vi "svx_Oct_Waterfall Shortcut Menu.vi"(7 "main graph?":bool, 9 "Container State":T2, 10 "State":T1, 11 "menu reference in":refnum<k9>) -> (3 "menu referenceout":refnum<k9>)   [LabVIEW 2017, in "SVX Octave Waterfall Graph.xctl"]
uses:
  <vilib>/addons/_XControls/Octave Waterfall Graph/SVX Octave Waterfall Graph.xctl
  <vilib>/_xctls/Container State.ctl
  <vilib>/addons/_XControls/Octave Waterfall Graph/subVIs/svx_Oct_Waterfall State.ctl
  <vilib>/_xctls/XControlSupport.lvlib
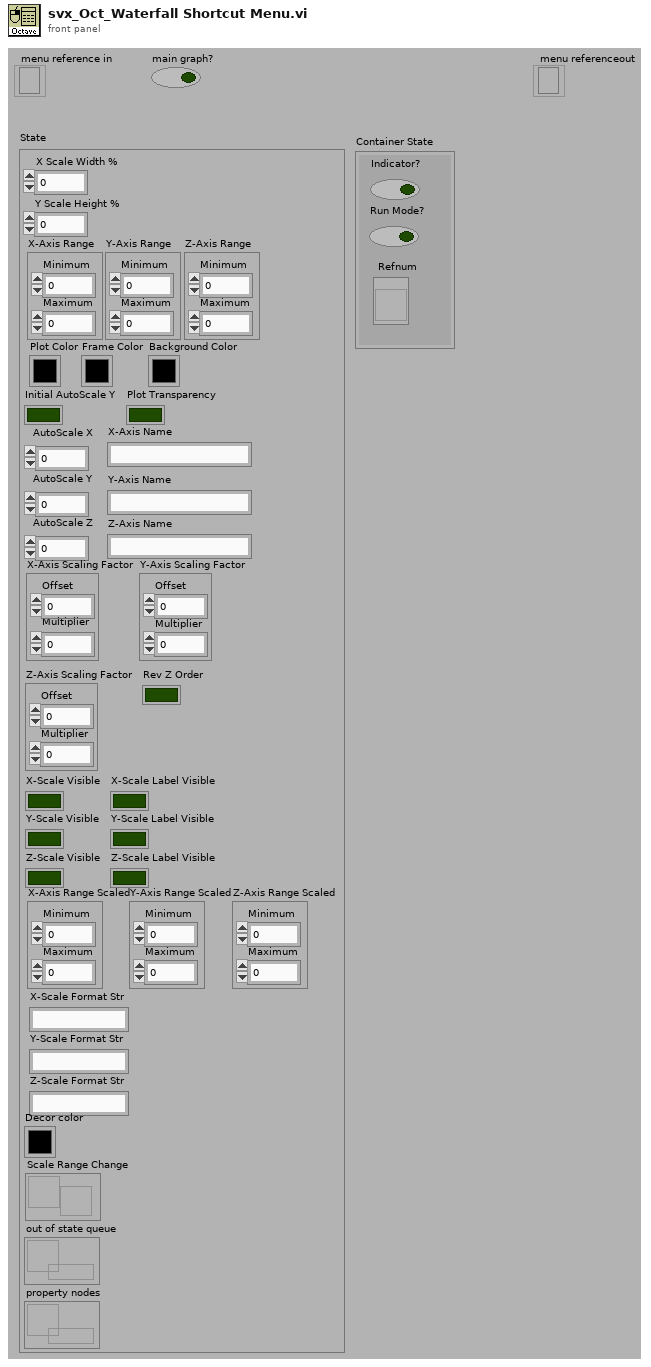
[diagram p1: front panel]
types:
  T1 = typedef "SVX Octave Waterfall Graph.xctl/svx_Oct_Waterfall State.ctl" = cluster{"X Scale Width %":dbl, "Y Scale Height %":dbl, "X-Axis Range":cluster{"Minimum":dbl, "Maximum":dbl}, "Y-Axis Range":cluster{"Minimum":dbl, "Maximum":dbl}, "Z-Axis Range":cluster{"Minimum":dbl, "Maximum":dbl}, "Plot Color":u32, "Frame Color":u32, "Background Color":u32, "Initial AutoScale Y":bool, "AutoScale X":u8, "AutoScale Y":u8, "AutoScale Z":u8, "Plot Transparency":bool, "X-Axis Name":string, "Y-Axis Name":string, "Z-Axis Name":string, "X-Axis Scaling Factor":cluster{"Offset":dbl, "Multiplier":dbl}, "Y-Axis Scaling Factor":cluster{"Offset":dbl, "Multiplier":dbl}, "Z-Axis Scaling Factor":cluster{"Offset":dbl, "Multiplier":dbl}, "X-Scale Visible":bool, "Y-Scale Visible":bool, "Z-Scale Visible":bool, "X-Scale Label Visible":bool, "Y-Scale Label Visible":bool, "Z-Scale Label Visible":bool, "X-Axis Range Scaled":cluster{"Minimum":dbl, "Maximum":dbl}, "Y-Axis Range Scaled":cluster{"Minimum":dbl, "Maximum":dbl}, "Z-Axis Range Scaled":cluster{"Minimum":dbl, "Maximum":dbl}, "Rev Z Order":bool, "X-Scale Format Str":string, "Y-Scale Format Str":string, "Z-Scale Format Str":string, "Decor color":u32, "Scale Range Change":refnum<user-event>, "out of state queue":refnum<queue>, "property nodes":refnum<queue>}
  T2 = typedef "XControlSupport.lvlib/Container State.ctl" = cluster{"Indicator?":bool, "Run Mode?":bool, " Refnum":refnum<vi>}
  T3 = cluster{"menu tag":string, "items to delete":string[], "new menu":cluster{"item names":string, "item tags":string, "after item":string}[], "root?":bool}
  T4 = cluster{"menu tag":string, "items to delete":string[], "new menu":cluster{"item names":string, "item tags":string, "after item":string}[], "root?":bool}[]
  T5 = cluster{"item names":string, "item tags":string, "after item":string}[]
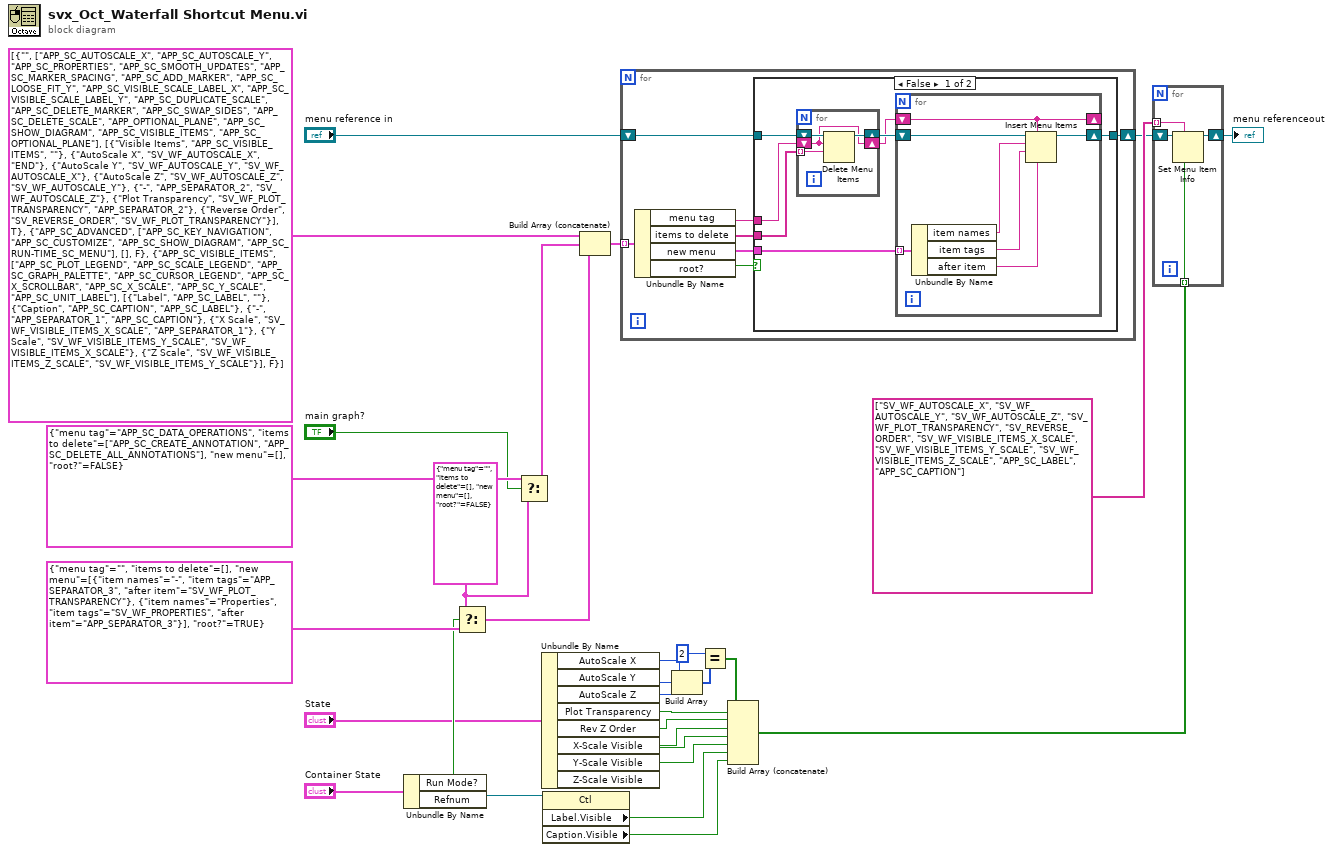
[diagram p0: block diagram]
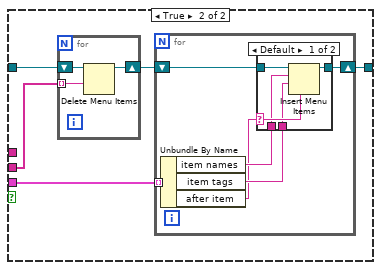
[diagram p2: hidden frame]
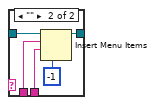
[diagram p3: hidden frame]
diagram:
  w27 = T3 {"menu tag"="", "items to delete"=[], "new menu"=[], "root?"=FALSE} ("t")
  n1 = Unbundle By Name("Container State") -> ("Run Mode?"=w6:bool, "Refnum"=w20:refnum<vi>)
  n2 = Select(t=w27, s=w6, f=T3 {"menu tag"="", "items to delete"=[], "new menu"=[{"item names"="-", "item tags"="APP_SEPARATOR_3", "after item"="SV_WF_PLOT_TRANSPARENCY"}, {"item names"="Properties", "item tags"="SV_WF_PROPERTIES", "after item"="APP_SEPARATOR_3"}], "root?"=TRUE} ("menu item")) -> (s? t:f=w24:T3)
  n3 = Select(t=T3 {"menu tag"="APP_SC_DATA_OPERATIONS", "items to delete"=["APP_SC_CREATE_ANNOTATION", "APP_SC_DELETE_ALL_ANNOTATIONS"], "new menu"=[], "root?"=FALSE} ("menu item"), s="main graph?", f=w27) -> (s? t:f=w25:T3)
  n4 = Unbundle By Name("State") -> ("AutoScale X"=w15:u8, "AutoScale Y"=w16:u8, "AutoScale Z"=w13:u8, "Plot Transparency"=w3:bool, "Rev Z Order"=w2:bool, "X-Scale Visible"=w17:bool, "Y-Scale Visible"=w18:bool, "Z-Scale Visible"=w19:bool)
  n5 = property class="Ctl"(reference=w20) -> ("Label.Visible"=w21:bool, "Caption.Visible"=w22:bool)  [unwired: 1 in, 2 out]
  n6 = Build Array (concatenate)(T4 [{"menu tag"="", "items to delete"=["APP_SC_AUTOSCALE_X", "APP_SC_AUTOSCALE_Y", "APP_SC_PROPERTIES", "APP_SC_SMOOTH_UPDATES", "APP_SC_MARKER_SPACING", "APP_SC_ADD_MARKER", "APP_SC_LOOSE_FIT_Y", "APP_SC_VISIBLE_SCALE_LABEL_X", "APP_SC_VISIBLE_SCALE_LABEL_Y", "APP_SC_DUPLICATE_SCALE", "APP_SC_DELETE_MARKER", "APP_SC_SWAP_SIDES", "APP_SC_DELETE_SCALE", "APP_OPTIONAL_PLANE", "APP_SC_SHOW_DIAGRAM", "APP_SC_VISIBLE_ITEMS", "APP_SC_OPTIONAL_PLANE"], "new menu"=[{"item names"="Visible Items", "item tags"="APP_SC_VISIBLE_ITEMS", "after item"=""}, {"item names"="AutoScale X", "item tags"="SV_WF_AUTOSCALE_X", "after item"="END"}, {"item names"="AutoScale Y", "item tags"="SV_WF_AUTOSCALE_Y", "after item"="SV_WF_AUTOSCALE_X"}, {"item names"="AutoScale Z", "item tags"="SV_WF_AUTOSCALE_Z", "after item"="SV_WF_AUTOSCALE_Y"}, {"item names"="-", "item tags"="APP_SEPARATOR_2", "after item"="SV_WF_AUTOSCALE_Z"}, {"item names"="Plot Transparency", "item tags"="SV_WF_PLOT_TRANSPARENCY", "after item"="APP_SEPARATOR_2"}, {"item names"="Reverse Order", "item tags"="SV_REVERSE_ORDER", "after item"="SV_WF_PLOT_TRANSPARENCY"}], "root?"=TRUE}, {"menu tag"="APP_SC_ADVANCED", "items to delete"=["APP_SC_KEY_NAVIGATION", "APP_SC_CUSTOMIZE", "APP_SC_SHOW_DIAGRAM", "APP_SC_RUN-TIME_SC_MENU"], "new menu"=[], "root?"=FALSE}, {"menu tag"="APP_SC_VISIBLE_ITEMS", "items to delete"=["APP_SC_PLOT_LEGEND", "APP_SC_SCALE_LEGEND", "APP_SC_GRAPH_PALETTE", "APP_SC_CURSOR_LEGEND", "APP_SC_X_SCROLLBAR", "APP_SC_X_SCALE", "APP_SC_Y_SCALE", "APP_SC_UNIT_LABEL"], "new menu"=[{"item names"="Label", "item tags"="APP_SC_LABEL", "after item"=""}, {"item names"="Caption", "item tags"="APP_SC_CAPTION", "after item"="APP_SC_LABEL"}, {"item names"="-", "item tags"="APP_SEPARATOR_1", "after item"="APP_SC_CAPTION"}, {"item names"="X Scale", "item tags"="SV_WF_VISIBLE_ITEMS_X_SCALE", "after item"="APP_SEPARATOR_1"}, {"item names"="Y Scale", "item tags"="SV_WF_VISIBLE_ITEMS_Y_SCALE", "after item"="SV_WF_VISIBLE_ITEMS_X_SCALE"}, {"item names"="Z Scale", "item tags"="SV_WF_VISIBLE_ITEMS_Z_SCALE", "after item"="SV_WF_VISIBLE_ITEMS_Y_SCALE"}], "root?"=FALSE}] ("edit-time menu"), w25, w24) -> (w23:T4)
  n7 = for {
    tunnel: w23 -> [w37] mode=indexing
    shift-right: [w32] -> w9
    shift-left: "menu reference in" -> [w36]
    n8 = Unbundle By Name(w37) -> ("menu tag"=w35:string, "items to delete"=w34:string[], "new menu"=w33:T5, "root?"=w31:bool)
    n9 = case shown="False" w31 {
      tunnel: w36 -> [w44 w60]
      tunnel: w35 -> [w43 _]
      tunnel: w34 -> [w42 w59]
      tunnel: w33 -> [w39 w57]
      tunnel: [w38 w56] -> w32
      frame False {
        n10 = for {
          shift-right: [w54] -> w41
          shift-left: w44 -> [w55]
          shift-right: [w52] -> w40
          shift-left: w43 -> [w52]
          tunnel: w42 -> [w53] mode=indexing
          n11 = Delete Menu Items(7:w53, 8:w52, 9:w55) -> (3:w54:refnum<k9>)  [unwired: 1 in, 1 out]
        }
        n12 = for {
          shift-right: [w45] -> w38
          shift-left: w41 -> [w51]
          shift-right: [w50] -> _
          shift-left: w40 -> [w50]
          tunnel: w39 -> [w49] mode=indexing
          n13 = Unbundle By Name(w49) -> ("item names"=w48:string, "item tags"=w47:string, "after item"=w46:string)
          n14 = Insert Menu Items(4:w46, 5:w50, 7:w47, 8:w48, 9:w51) -> (3:w45:refnum<k9>)  [unwired: 1 in, 2 out]
        }
      }
      frame True {
        n15 = for {
          shift-right: [w78] -> w58
          shift-left: w60 -> [w79]
          tunnel: w59 -> [w77] mode=indexing
          n16 = Delete Menu Items(7:w77, 9:w79) -> (3:w78:refnum<k9>)  [unwired: 2 in, 1 out]
        }
        n17 = for {
          shift-right: [w66] -> w56
          shift-left: w58 -> [w65]
          tunnel: w57 -> [w64] mode=indexing
          n18 = Unbundle By Name(w64) -> ("item names"=w63:string, "item tags"=w62:string, "after item"=w61:string)
          n19 = case shown="Default" w61 {
            selector: w61 -> [w69 _]
            tunnel: [w70 w76] -> w66
            tunnel: w65 -> [w71 w75]
            tunnel: w63 -> [w68 w74]
            tunnel: w62 -> [w67 w73]
            frame Default {
              n20 = Insert Menu Items(4:w69, 7:w67, 8:w68, 9:w71) -> (3:w70:refnum<k9>)  [unwired: 2 in, 2 out]
            }
            frame "" {
              n21 = Insert Menu Items(4:-1, 7:w73, 8:w74, 9:w75) -> (3:w76:refnum<k9>)  [unwired: 2 in, 2 out]
            }
          }
        }
      }
    }
  }
  n22 = Build Array(w15, w16, w13) -> (w14:u8[])
  n23 = Equal?(x=u8 2 ("y"), y=w14) -> (x = y?=w4:bool[])
  n24 = Build Array (concatenate)(w4, w3, w2, w17, w18, w19, w21, w22) -> (w8:bool[])
  n25 = for {
    tunnel: string[] ["SV_WF_AUTOSCALE_X", "SV_WF_AUTOSCALE_Y", "SV_WF_AUTOSCALE_Z", "SV_WF_PLOT_TRANSPARENCY", "SV_REVERSE_ORDER", "SV_WF_VISIBLE_ITEMS_X_SCALE", "SV_WF_VISIBLE_ITEMS_Y_SCALE", "SV_WF_VISIBLE_ITEMS_Z_SCALE", "APP_SC_LABEL", "APP_SC_CAPTION"] -> [w83] mode=indexing
    tunnel: w8 -> [w81] mode=indexing
    shift-right: [w80] -> w7
    shift-left: w9 -> [w82]
    n26 = Set Menu Item Info(6:w81, 7:w83, 11:w82) -> (3:w80:refnum<k9>)  [unwired: 4 in, 1 out]
  }
  "menu referenceout" <- w7
